vi "Android Deploy.vi"() -> ()   [LabVIEW 2016]
uses:
  Constants/Typedef/Constants.ctl
  <vilib>/Rock Robotics/SystemInterfaces/DIO/FPGA_DIOPWMChannel.ctl
  <vilib>/Rock Robotics/WPI/Joystick/WPI_JoystickDeviceEnum.ctl
  <vilib>/Rock Robotics/SystemInterfaces/DIO/FPGA_DIOChannel.ctl
  <vilib>/Rock Robotics/SystemInterfaces/spilib/spi_bus.ctl
  <vilib>/Rock Robotics/SystemInterfaces/AI/FPGA_AIChannel.ctl
  <vilib>/Rock Robotics/WPI/Solenoid/WPI_SolenoidChannel.ctl
  Constants/Constants.lvlib
panel:
  in  "Set As Defaults":bool
  in  "Generate Constants File":bool
  in  "Constants xml":path caption="Constants File"
  in  "Host":string="172.22.11.2"
  in  "Clear Cache":bool
  in  "Clear":bool
  out "Console":string
  in  "RIOdroid Directory":path caption="RIOdroid Directory (Includes RIOdroid.tar.gz and RIOdroid.roborio.sh)"
  in  "Setup RIO":bool
  in  "Andoid APK App":path
  in  "Load APK":bool
  # "Android Vision App - Deploy Tools"
  # "Fix target failed to deploy with errors issue by clearing the object cache."
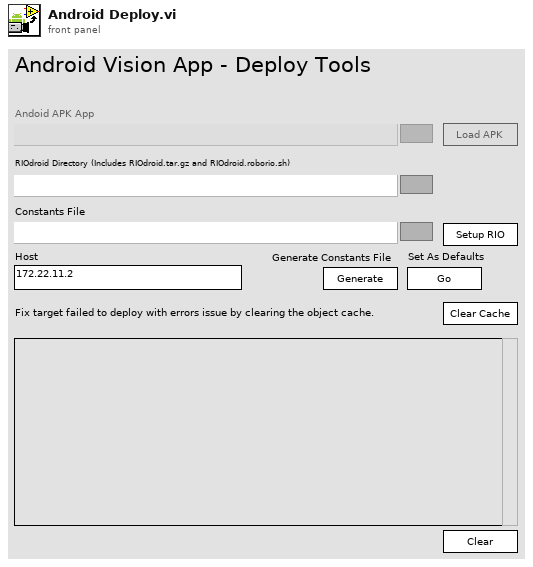
[diagram p1: front panel]
types:
  T1 = cluster{"plink":path, "pscp":path, "Console":refnum<vi>}
  T2 = typedef "Constants.lvlib/Constants.ctl" = cluster{"Port Layout":cluster{"RightMotorInverted":bool, "LeftMotorInverted":bool, "Left Motors":T3, "Right Motors":T3, "Auton List":string[], "XBOX Port":T4, "Encoder L A":T5, "Encoder L B":T5, "Encoder R A":T5, "Encoder R B":T5, "L Encoder Inverse":bool, "R Encoder Inverse":bool, "Drive Distance per Count":dbl, "Gyro Bus":T6, "Fuel Roller 1":T3, "Front Roller":T3, "Gear Flipper":T3, "Climber 1":T3, "Fuel Roller Invert":bool, "Front Roller Invert":bool, "Gear Flipper Invert":bool, "Climber Invert":bool, "PCM":u8, "Fuel Roller 2":T3, "Gear Sensor":T7, "Gear Release Fwd":T8, "Gear Release Rvrs":T8, "Fuel Arm Fwd":T8, "Fuel Arm Rvrs":T8, "Shifter Fwrd":T8, "Shifter Rvrs":T8, "Climber 2":T3, "PDP":u8, "Shooter Front Channel":u8, "Shooter Rear Channel":u8, "Shooter Feed Channel":u8, "Camera Servo":T3, "Gear Servo":T3, "Gear Puncher Fwrd":T8, "Gear Puncher Rvrs":T8, "Shooter Inverse":bool, "Ring Light Switch":T5}, "Drive Constants":cluster{"Wheelbase In.":dbl, "Max Velocity (In/sec)":dbl, "Max Accel (In/sec^2)":dbl, "Max Jerk (In/sec^3)":dbl, "Path dt":dbl, "Path Sample Count":i32, "Deadband":dbl}, "Arm System":cluster{"Front Roller Gear Speed":dbl, "Front Roller Fuel Speed":dbl, "Gear Flipper Speed":dbl, "Fuel Roller Speed":dbl, "Gear Release Wait (ms)":i32, "Gear Sensor Threshold":dbl, "Flappy Open Angle":i32, "Flappy Close Angle":i32, "Ramp Rate (EGU/min)":dbl}, "Shooter":cluster{"Shooter Wheels":cluster{"P":dbl, "I":dbl, "D":dbl, "F":dbl, "IZone":dbl}, "Feeder":cluster{"P":dbl, "I":dbl, "D":dbl, "F":dbl, "IZone":dbl}, "Front Shooter RPM":dbl, "Rear Shooter RPM":dbl, "Agitator Speed":dbl, "Feeder Speed":dbl, "Shooter CPR":u32, "Feeder CPR":u32}, "Vision":cluster{"High Goal Height (in.)":dbl, "Low Goal Height (in.)":dbl, "Camera Height High (in.)":dbl, "Camera Height Low (in.)":dbl, "Servo Pitch Gear (deg)":dbl, "Camera Yaw (deg)":dbl, "Servo Gear":i32, "Servo Boiler":i32, "Servo Pitch Boiler (deg)":dbl}}
  T3 = typedef "FPGA_DIOPWMChannel.ctl" = enum8{"PWM 0", "PWM 1", "PWM 2", "PWM 3", "PWM 4", "PWM 5", "PWM 6", "PWM 7", "PWM 8", "PWM 9", "PWM MXP 0", "PWM MXP 1", "PWM MXP 2", "PWM MXP 3", "PWM MXP 4", "PWM MXP 5", "PWM MXP 6", "PWM MXP 7", "PWM MXP 8", "PWM MXP 9", "Invalid"}
  T4 = typedef "WPI_JoystickDeviceEnum.ctl" = enum16{"USB 0", "USB 1", "USB 2", "USB 3", "USB 4", "USB 5"}
  T5 = typedef "FPGA_DIOChannel.ctl" = enum8{"DIO 0", "DIO 1", "DIO 2", "DIO 3", "DIO 4", "DIO 5", "DIO 6", "DIO 7", "DIO 8", "DIO 9", "DIO MXP 0", "DIO MXP 1", "DIO MXP 2", "DIO MXP 3", "DIO MXP 4", "DIO MXP 5", "DIO MXP 6", "DIO MXP 7", "DIO MXP 8", "DIO MXP 9", "DIO MXP 10", "DIO MXP 11", "DIO MXP 12", "DIO MXP 13", "DIO MXP 14", "DIO MXP 15", "SPI Port CS1", "SPI Port CS2", "SPI Port CS3", "SPI Port MISO", "SPI Port MOSI", "Invalid"}
  T6 = typedef "spi_bus.ctl" = enum16{"SPI On-Board, CS0", "SPI On-Board, CS1", "SPI On-Board, CS2", "SPI On-Board, CS3", "SPI MXP", "Invalid"}
  T7 = typedef "FPGA_AIChannel.ctl" = enum8{"AI 0", "AI 1", "AI 2", "AI 3", "AI MXP 0", "AI MXP 1", "AI MXP 2", "AI MXP 3", "Invalid"}
  T8 = typedef "WPI_SolenoidChannel.ctl" = enum8{"Solenoid 0", "Solenoid 1", "Solenoid 2", "Solenoid 3", "Solenoid 4", "Solenoid 5", "Solenoid 6", "Solenoid 7", "Invalid"}
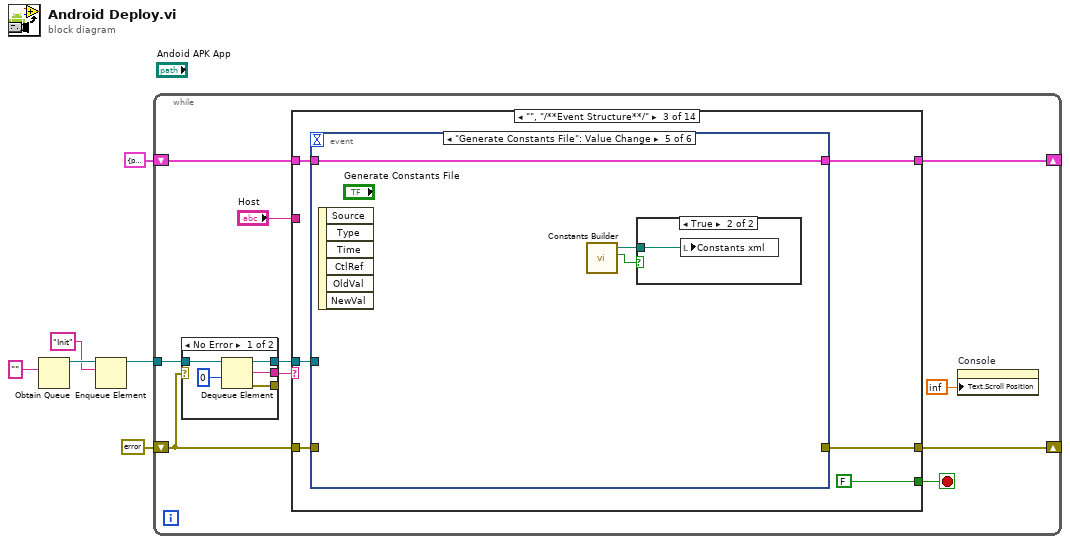
[diagram p0: block diagram]
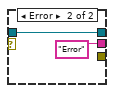
[diagram p2: hidden frame]
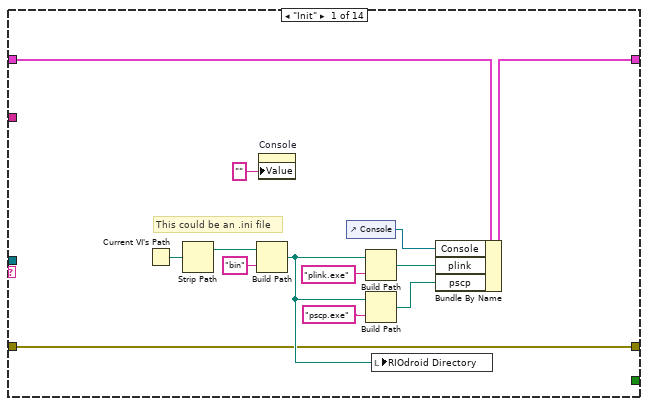
[diagram p3: hidden frame]
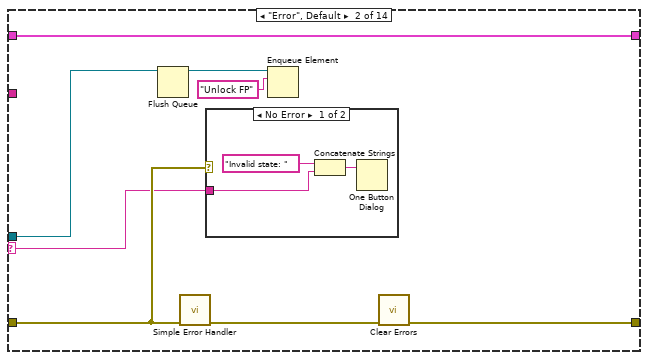
[diagram p4: hidden frame]
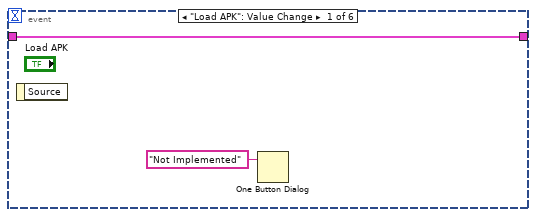
[diagram p6: hidden frame]
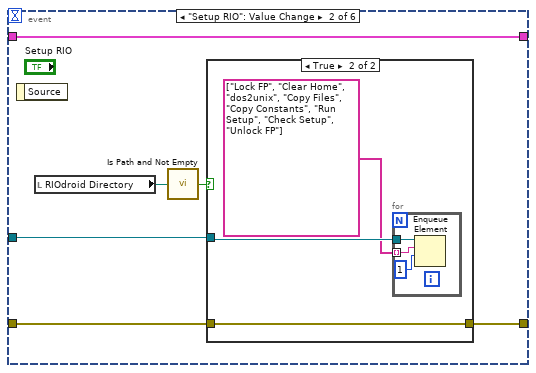
[diagram p7: hidden frame]
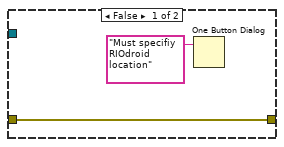
[diagram p8: hidden frame]
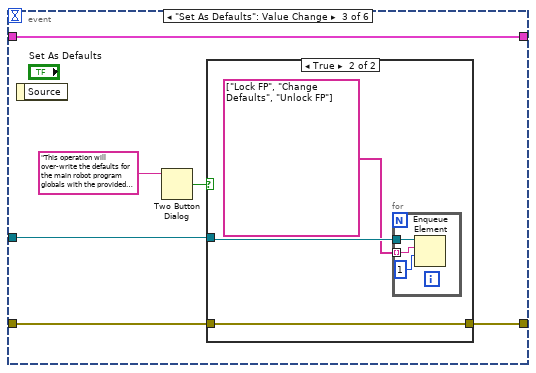
[diagram p9: hidden frame]
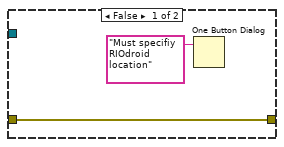
[diagram p10: hidden frame]
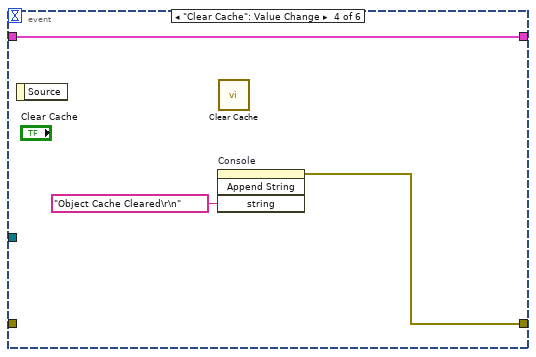
[diagram p11: hidden frame]
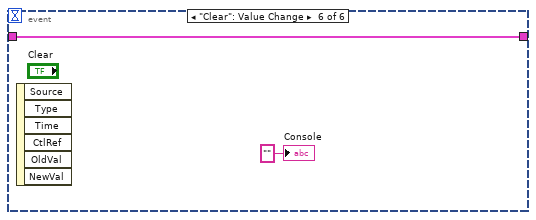
[diagram p13: hidden frame]
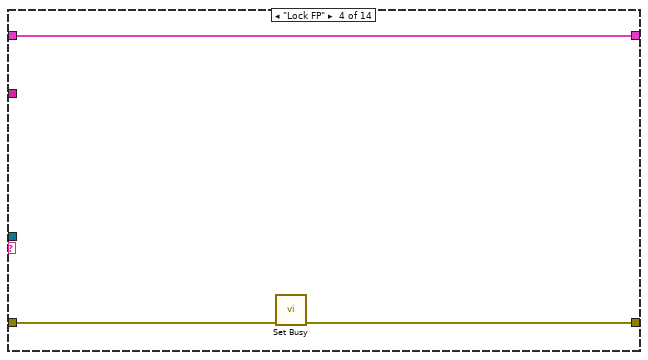
[diagram p14: hidden frame]
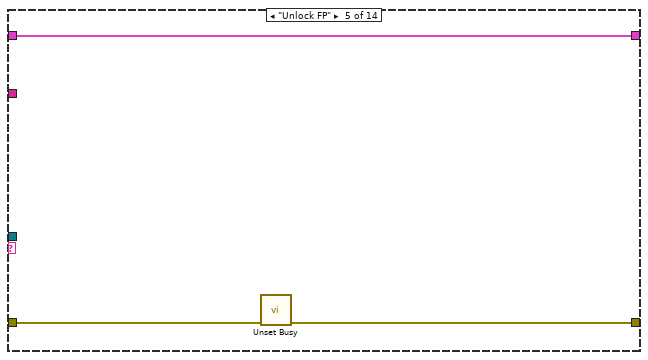
[diagram p15: hidden frame]
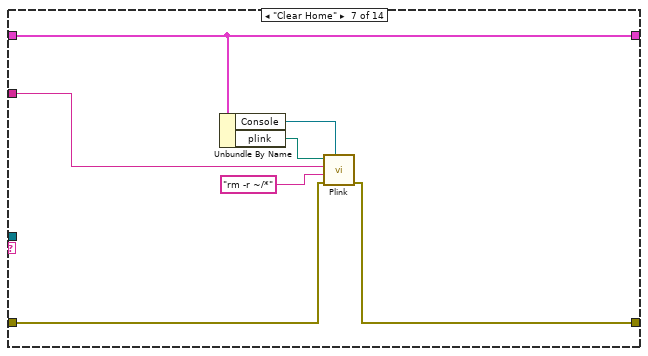
[diagram p17: hidden frame]
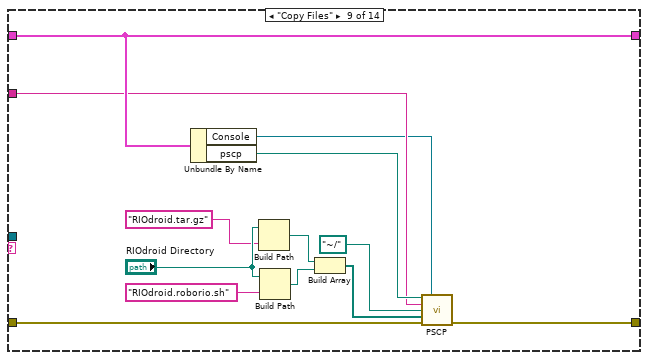
[diagram p19: hidden frame]
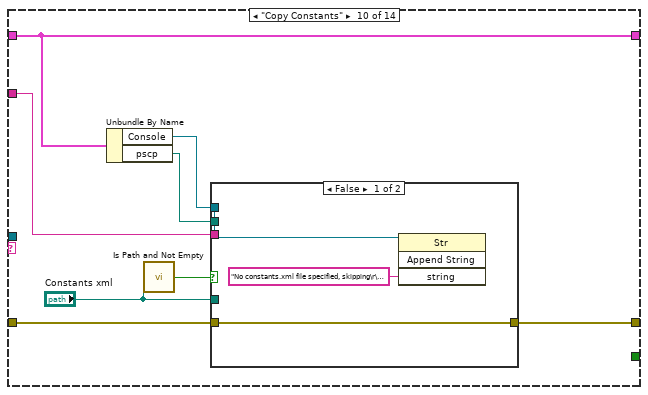
[diagram p20: hidden frame]
diagram:
  n1 = Obtain Queue(element data type="" ("Console")) -> (queue out=w5:refnum<queue>)  [unwired: 4 in, 2 out]
  n2 = Enqueue Element(queue=w5, element="Init") -> (queue out=w4:refnum<queue>)  [unwired: 2 in, 2 out]
  n3 = while {
    tunnel: w4 -> [w15]
    shift-right: [w12] -> _
    shift-left: T1 {"plink"=path "", "pscp"=path "", "Console"=refnum} -> [w13]
    shift-right: [w10] -> _
    shift-left: errorcluster {"status"=FALSE, "code"=0, "source"=""} ("error out") -> [w7]
    stop <- w14 stop-if-true
    n4 = case shown="No Error" w7 {
      tunnel: [w21 "Error" ("Console")] -> w16
      tunnel: w15 -> [w20 w23]
      tunnel: [w18 w23] -> w8
      tunnel: [w17 _] -> _
      frame No Error {
        n5 = Dequeue Element(queue=w20, timeout in ms (-1)=0) -> (queue out=w18:refnum<queue>, element=w21:string, error out=w17:errorcluster)  [unwired: 1 in, 1 out]
      }
      frame Error {
      }
    }
    n6 = case shown="\"\", \"/**Event Structure**/\"" w16 {
      selector: w16 -> [_ w40 _ _ _ _ _ _ _ _ _ _ _ _]
      tunnel: [_ _ FALSE _ _ _ _ _ _ _ _ _ _ _] -> w14
      tunnel: [w24 w42 w48 w93 w96 w99 w102 w108 w121 w129 w144 w160 w166 w169] -> w10
      tunnel: w13 -> [w30 w44 w52 w95 w98 w100 w105 w109 w118 w128 w147 w163 w167 w178]
      tunnel: [w29 w44 w51 w95 w98 w100 w105 w109 w118 w128 w147 w163 w167 w178] -> w12
      tunnel: "Host" -> [_ _ _ _ _ _ w106 _ w116 w126 w148 w164 _ _]
      tunnel: w7 -> [w24 w41 w49 w94 w97 w99 w103 w108 w122 w130 w145 w161 w166 w170]
      tunnel: w8 -> [_ w39 w50 _ _ _ _ _ _ _ _ _ _ _]
      frame "Init" {
        # "This could be an .ini file"
        n7 = Current VI's Path() -> (path=w31:path)
        n8 = Strip Path(path=w31) -> (stripped path=w32:path)  [unwired: 1 out]
        n9 = Build Path(base path=w32, name or relative path="bin") -> (appended path=w28:path)
        n10 = property on="Console" class="Str"("Value"="" ("Console")) -> ()  [unwired: 2 in, 2 out]
        n11 = control-ref of="Console"() -> (w25:refnum<vi>)
        n12 = Build Path(base path=w28, name or relative path="plink.exe") -> (appended path=w26:path)
        n13 = Build Path(base path=w28, name or relative path="pscp.exe") -> (appended path=w27:path)
        n14 = local write "RIOdroid Directory"(w28) -> ()
        n15 = Bundle By Name(cluster=w30, "Console"=w25, "plink"=w26, "pscp"=w27) -> (w29:T1)
      }
      frame "Error", Default {
        n16 = Flush Queue(queue=w39) -> (queue out=w38:refnum<queue>)  [unwired: 1 in, 2 out]
        n17 = call <vilib>:"Simple Error Handler.vi"("error in (no error)"=w41) -> ("error out"=w43:errorcluster)  [unwired: 4 in, 4 out]
        n18 = case shown="No Error" w41 {
          tunnel: w40 -> [w46 _]
          frame No Error {
            n19 = Concatenate Strings("Invalid state: " ("message"), w46) -> (w45:string)
            n20 = One Button Dialog(message=w45) -> ()  [unwired: 1 in, 1 out]
          }
          frame Error {
          }
        }
        n21 = Enqueue Element(queue=w38, element="Unlock FP") -> ()  [unwired: 2 in, 3 out]
        n22 = call <vilib>:"Clear Errors.vi"("error in (no error)"=w43) -> ("error out"=w42:errorcluster)  [unwired: 5 in, 1 out]
      }
      frame "", "/**Event Structure**/" {
        n23 = event shown="[4] \"Generate Constants File\": Value Change" {
          selector: _ -> [_ _ _ _ _ _]
          dyn-events: _ -> [_ _ _ _ _ _]
          timeout: _ -> [_ _ _ _ _ _]
          tunnel: w52 -> [w55 w61 w75 w85 w89 w91]
          tunnel: [w55 w61 w75 w85 w89 w91] -> w51
          tunnel: w50 -> [_ w56 w72 _ _ _]
          tunnel: w49 -> [_ w59 w74 _ _ _]
          tunnel: [_ w58 w73 w84 _ _] -> w48
          event "Load APK": Value Change {
            n24 = event-data() -> ()  [unwired: 1 in, 1 out]
            n25 = One Button Dialog(message="Not Implemented") -> ()  [unwired: 1 in, 1 out]
          }
          event "Setup RIO": Value Change {
            n26 = event-data() -> ()  [unwired: 1 in, 1 out]
            n27 = local read "RIOdroid Directory"() -> (w60:path)
            n28 = call <vilib>:"Is Path and Not Empty.vi"("path"=w60) -> ("Is Path and Not Empty?"=w57:bool)  [unwired: 4 in]
            n29 = case shown="True" w57 {
              tunnel: w59 -> [w63 w66]
              tunnel: [w63 w66] -> w58
              tunnel: w56 -> [_ w65]
              frame False {
                n30 = One Button Dialog(message="Must specifiy RIOdroid location") -> ()  [unwired: 1 in, 1 out]
              }
              frame True {
                n31 = for {
                  tunnel: w65 -> [w69]
                  tunnel: string[] ["Lock FP", "Clear Home", "dos2unix", "Copy Files", "Copy Constants", "Run Setup", "Check Setup", "Unlock FP"] -> [w68] mode=indexing
                  n32 = Enqueue Element(queue=w69, element=w68, timeout in ms (-1)=1) -> ()  [unwired: 1 in, 3 out]
                }
              }
            }
          }
          event "Set As Defaults": Value Change {
            n33 = event-data() -> ()  [unwired: 1 in, 1 out]
            n34 = Two Button Dialog(message="This operation will over-write the defaults for the main robot program globals with the provided xml, continue?") -> (T button?=w71:bool)  [unwired: 2 in]
            n35 = case shown="True" w71 {
              tunnel: w74 -> [w77 w80]
              tunnel: [w77 w80] -> w73
              tunnel: w72 -> [_ w79]
              frame False {
                n36 = One Button Dialog(message="Must specifiy RIOdroid location") -> ()  [unwired: 1 in, 1 out]
              }
              frame True {
                n37 = for {
                  tunnel: w79 -> [w83]
                  tunnel: string[] ["Lock FP", "Change Defaults", "Unlock FP"] -> [w82] mode=indexing
                  n38 = Enqueue Element(queue=w83, element=w82, timeout in ms (-1)=1) -> ()  [unwired: 1 in, 3 out]
                }
              }
            }
          }
          event "Clear Cache": Value Change {
            n39 = event-data() -> ()  [unwired: 1 in, 1 out]
            n40 = invoke on="Console" class="Str" method="Append String"("string"="Object Cache Cleared\r\n") -> (error out=w84:errorcluster)  [unwired: 3 in, 3 out]
            n41 = call "Clear Cache.vi"() -> ()  [unwired: 12 in]
          }
          event "Generate Constants File": Value Change {
            n42 = event-data() -> ()  [unwired: 1 in, 6 out]
            n43 = call "Constants Builder.vi"() -> ("Written?"=w87:bool, "path"=w88:path)  [unwired: 9 in, 1 out]
            n44 = case shown="True" w87 {
              tunnel: w88 -> [_ w90]
              frame False {
              }
              frame True {
                n45 = local write "Constants xml"(w90) -> ()
              }
            }
          }
          event "Clear": Value Change {
            n46 = event-data() -> ()  [unwired: 1 in, 6 out]
            "Console" <- "" ("Console")
          }
        }
      }
      frame "Lock FP" {
        n47 = call <vilib>:"Set Busy.vi"("error in (no error)"=w94) -> ("error out"=w93:errorcluster)  [unwired: 9 in, 1 out]
      }
      frame "Unlock FP" {
        n48 = call <vilib>:"Unset Busy.vi"("error in (no error)"=w97) -> ("error out"=w96:errorcluster)  [unwired: 10 in]
      }
      frame "/**Setup RIO States**/" {
      }
      frame "Clear Home" {
        n49 = Unbundle By Name(w105) -> ("Console"=w101:refnum<vi>, "plink"=w104:path)
        n50 = call "Plink.vi"("Console"=w101, "error in"=w103, "Command(s) to Execute"="rm -r ~/*", "Host"=w106, "plink path"=w104) -> ("error out"=w102:errorcluster)  [unwired: 2 in, 4 out]
      }
      frame "dos2unix" {
        # "Convert any text file from dos line endings to unix before sending"
      }
      frame "Copy Files" {
        n51 = Unbundle By Name(w118) -> ("Console"=w110:refnum<vi>, "pscp"=w117:path)
        n52 = Build Path(base path="RIOdroid Directory", name or relative path="RIOdroid.tar.gz") -> (appended path=w112:path)
        n53 = Build Path(base path="RIOdroid Directory", name or relative path="RIOdroid.roborio.sh") -> (appended path=w120:path)
        n54 = Build Array(w112, w120) -> (w115:path[])
        n55 = call "PSCP.vi"("pscp path"=w117, "Console"=w110, "Host"=w116, "remote path"=path "~/", "Files"=w115, "error in"=w122) -> ("error out"=w121:errorcluster)  [unwired: 5 in, 4 out]
      }
      frame "Copy Constants" {
        n56 = Unbundle By Name(w128) -> ("Console"=w125:refnum<vi>, "pscp"=w127:path)
        n57 = call <vilib>:"Is Path and Not Empty.vi"("path"="Constants xml") -> ("Is Path and Not Empty?"=w124:bool)  [unwired: 4 in]
        n58 = case shown="False" w124 {
          tunnel: w130 -> [w133 w142]
          tunnel: [w133 w141] -> w129
          tunnel: w127 -> [_ w140]
          tunnel: w126 -> [_ w139]
          tunnel: w125 -> [w132 w137]
          tunnel: "Constants xml" -> [_ w136]
          frame False {
            n59 = invoke class="Str" method="Append String"(reference=w132, "string"="No constants.xml file specified, skipping\r\n\r\n") -> ()  [unwired: 2 in, 4 out]
          }
          frame True {
            n60 = Build Array(w136) -> (w138:path[])
            n61 = String To Path(string="/home/lvuser/") -> (path=w134:path)
            n62 = call "PSCP.vi"("pscp path"=w140, "Console"=w137, "Host"=w139, "remote path"=w134, "Files"=w138, "error in"=w142) -> ("error out"=w141:errorcluster)  [unwired: 5 in, 4 out]
          }
        }
      }
      frame "Run Setup" {
        n63 = Unbundle By Name(w147) -> ("Console"=w143:refnum<vi>, "plink"=w146:path)
        n64 = call "Plink.vi"("Console"=w143, "error in"=w145, "Command(s) to Execute"="chmod +x ./RIOdroid.roborio.sh; ./RIOdroid.roborio.sh", "Host"=w148, "plink path"=w146) -> ("error out"=w144:errorcluster)  [unwired: 2 in, 4 out]
      }
      frame "Check Setup" {
        n65 = Unbundle By Name(w163) -> ("Console"=w159:refnum<vi>, "plink"=w162:path)
        n66 = invoke class="Str" method="Append String"(reference=w159, "string"="Running check for adb...\r\n\r\n") -> (reference out=w150:refnum<vi>)  [unwired: 2 in, 3 out]
        n67 = call "Plink.vi"("Console"=w150, "error in"=w161, "Command(s) to Execute"="adb devices; adb version", "Host"=w164, "plink path"=w162) -> ("error out"=w160:errorcluster, "Command Return Value(s)"=w157:string)  [unwired: 2 in, 3 out]
        n68 = Search and Replace String(input string=w157, search string="Android Debug Bridge") -> (offset past replacement=w155:i32)  [unwired: 6 in, 3 out]
        n69 = Less Than 0?(x=w155) -> (x < 0?=w154:bool)
        n70 = Select(t="ADB found and running" ("search string"), s=w154, f="ADB install not found!" ("search string")) -> (s? t:f=w151:string)
        n71 = invoke class="Str" method="Append String"(reference=w150, "string"=w151) -> ()  [unwired: 2 in, 4 out]
      }
      frame "/**Change Defaults Fcns**/" {
      }
      frame "Change Defaults" {
        n72 = local read "Constants xml"() -> (w168:path)
        n73 = Read from Text File(file (use dialog)=w168, error in=w170) -> (refnum out=w174:refnum<file>, text=w173:string, error out=w175:errorcluster)  [unwired: 2 in, 1 out]
        n74 = Close File(refnum=w174, error in=w175) -> (error out=w176:errorcluster)  [unwired: 1 out]
        n75 = Unflatten From XML(xml string=w173, type=T2 {"Port Layout"={"RightMotorInverted"=FALSE, "LeftMotorInverted"=TRUE, "Left Motors"=enum."PWM 0", "Right Motors"=enum."PWM 1", "Auton List"=["Alternative 1", "Alternative 2"], "XBOX Port"=enum."USB 0", "Encoder L A"=enum."DIO 3", "Encoder L B"=enum."DIO 4", "Encoder R A"=enum."DIO 5", "Encoder R B"=enum."DIO 6", "L Encoder Inverse"=FALSE, "R Encoder Inverse"=TRUE, "Drive Distance per Count"=1.0, "Gyro Bus"=enum."SPI On-Board, CS2", "Fuel Roller 1"=enum."PWM 0", "Front Roller"=enum."PWM 0", "Gear Flipper"=enum."PWM 0", "Climber 1"=enum."PWM 0", "Fuel Roller Invert"=TRUE, "Front Roller Invert"=TRUE, "Gear Flipper Invert"=TRUE, "Climber Invert"=TRUE, "PCM"=0, "Fuel Roller 2"=enum."PWM 0", "Gear Sensor"=enum."AI 0", "Gear Release Fwd"=enum."Solenoid 0", "Gear Release Rvrs"=enum."Solenoid 0", "Fuel Arm Fwd"=enum."Solenoid 0", "Fuel Arm Rvrs"=enum."Solenoid 0", "Shifter Fwrd"=enum."Solenoid 0", "Shifter Rvrs"=enum."Solenoid 0", "Climber 2"=enum."PWM 0", "PDP"=60, "Shooter Front Channel"=0, "Shooter Rear Channel"=0, "Shooter Feed Channel"=0, "Camera Servo"=enum."PWM 0", "Gear Servo"=enum."PWM 0", "Gear Puncher Fwrd"=enum."Solenoid 0", "Gear Puncher Rvrs"=enum."Solenoid 0", "Shooter Inverse"=TRUE, "Ring Light Switch"=enum."DIO 4"}, "Drive Constants"={"Wheelbase In."=1.0, "Max Velocity (In/sec)"=78.0, "Max Accel (In/sec^2)"=78.0, "Max Jerk (In/sec^3)"=0.0, "Path dt"=0.0, "Path Sample Count"=0, "Deadband"=0.35}, "Arm System"={"Front Roller Gear Speed"=0.8, "Front Roller Fuel Speed"=0.8, "Gear Flipper Speed"=0.8, "Fuel Roller Speed"=0.8, "Gear Release Wait (ms)"=1000, "Gear Sensor Threshold"=0.3, "Flappy Open Angle"=0, "Flappy Close Angle"=0, "Ramp Rate (EGU/min)"=200.0}, "Shooter"={"Shooter Wheels"={"P"=0.0, "I"=0.0, "D"=0.0, "F"=0.0, "IZone"=0.0}, "Feeder"={"P"=0.0, "I"=0.0, "D"=0.0, "F"=0.0, "IZone"=0.0}, "Front Shooter RPM"=0.0, "Rear Shooter RPM"=0.0, "Agitator Speed"=0.0, "Feeder Speed"=0.0, "Shooter CPR"=0, "Feeder CPR"=0}, "Vision"={"High Goal Height (in.)"=0.0, "Low Goal Height (in.)"=0.0, "Camera Height High (in.)"=0.0, "Camera Height Low (in.)"=0.0, "Servo Pitch Gear (deg)"=0.0, "Camera Yaw (deg)"=0.0, "Servo Gear"=0, "Servo Boiler"=0, "Servo Pitch Boiler (deg)"=0.0}} ("Constants"), error in (no error)=w176) -> (value=w171:T2, error out=w172:errorcluster)
        n76 = case shown="No Error" w172 {
          selector: w172 -> [w181 w183]
          tunnel: w171 -> [w182 _]
          tunnel: [w180 w183] -> w169
          frame No Error {
            n77 = call "Get Private Global Path.vi"() -> ("appended path"=w179:path)  [unwired: 11 in]
            n78 = call "Set Constants Default.vi"("error in (no error)"=w181, "Constants"=w182, "selected path"=w179) -> ("error out"=w180:errorcluster)  [unwired: 8 in]
          }
          frame Error {
          }
        }
      }
    }
    n79 = property on="Console" class="Str"("Text.Scroll Position"=inf) -> ()  [unwired: 2 in, 2 out]
  }
